vi "Read Message.vi"(8 "error in (no error)":errorcluster, 11 "Sender Msg in":refnum<class "Sender Msg.lvclass">) -> (0 "error out":errorcluster, 2 "Message":refnum<class "Message.lvclass">, 3 "Sender Msg out":refnum<class "Sender Msg.lvclass">)   [LabVIEW 2020, in "Publisher.lvlib" / "Sender Msg.lvclass"]
doc: "Read the message contained in the Sender Msg class."
uses:
  Sender Msg.lvclass
  PPL/HDH.Actor Framework.Core.Actor.lvlibp/1abvi3w/vi.lib/ActorFramework/Message/Message.lvclass
  Sender Msg.lvclass/Sender Msg.ctl
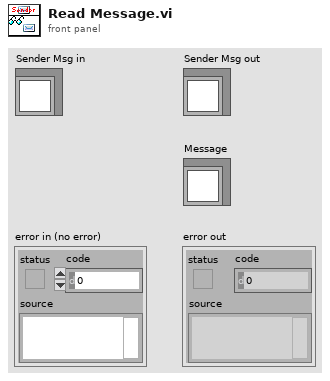
[diagram p1: front panel]
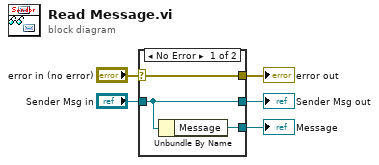
[diagram p0: block diagram]
diagram:
  n1 = case shown="No Error" "error in (no error)" {
    selector: "error in (no error)" -> [w8 w9]
    tunnel: [w8 w9] -> w4
    tunnel: [w7 w10] -> w2
    tunnel: "Sender Msg in" -> [w7 w10]
    tunnel: [w6 _] -> w1
    frame No Error {
      n2 = Unbundle By Name(w7) -> ("Message"=w6:refnum<class "Message.lvclass">)
    }
    frame Error {
    }
  }
  "error out" <- w4
  "Sender Msg out" <- w2
  "Message" <- w1
